vi "SetOpenedChannels.vi"(7 "Slot":T1, 8 "Error In":errorcluster, 9 "All?":bool, 10 "Channels":bool[](array[boolean]), 11 "Keithley 7001 In":refnum<visa-resource-name>) -> (0 "Error Out":errorcluster, 3 "Keithley 7001 Out":refnum<visa-resource-name>)   [LabVIEW 2012, in "Keithley-7001.lvlib"]
uses:
  Keithley-7001.lvlib
  Controls/Slot.ctl
panel:
  # "33"
  # "34"
  # "35"
  # "1"
  # "2"
  # "3"
  # "4"
  # "5"
  # "6"
  # "7"
  # "8"
  # "9"
  # "10"
  # "11"
  # "12"
  # "13"
  # "14"
  # "15"
  # "16"
  # "17"
  # "18"
  # "19"
  # "20"
  # "21"
  # "22"
  # "23"
  # "24"
  # "25"
  # "26"
  # "27"
  # "28"
  # "29"
  # "30"
  # "31"
  # "32"
  # "36"
  # "37"
  # "38"
  # "39"
  # "40"
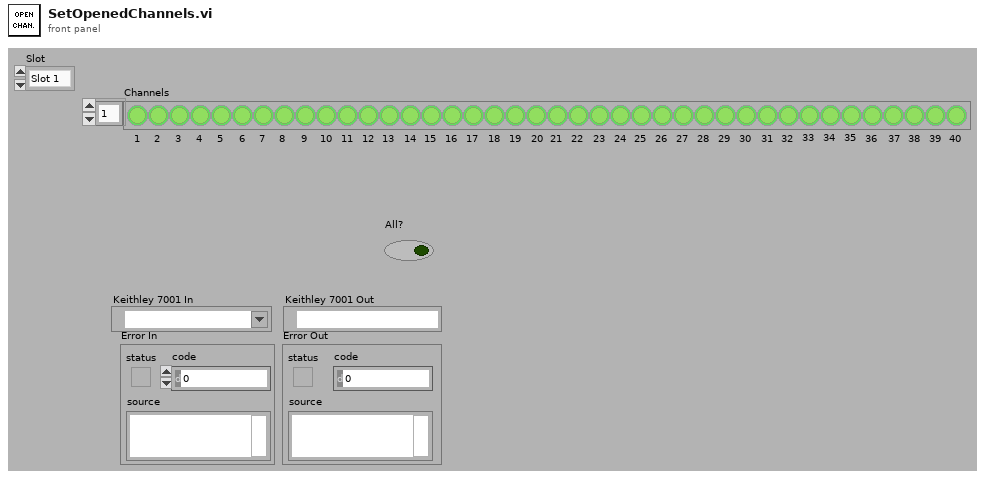
[diagram p1: front panel]
types:
  T1 = typedef "Keithley-7001.lvlib/Slot.ctl" = enum16{"Slot 1", "Slot 2"}
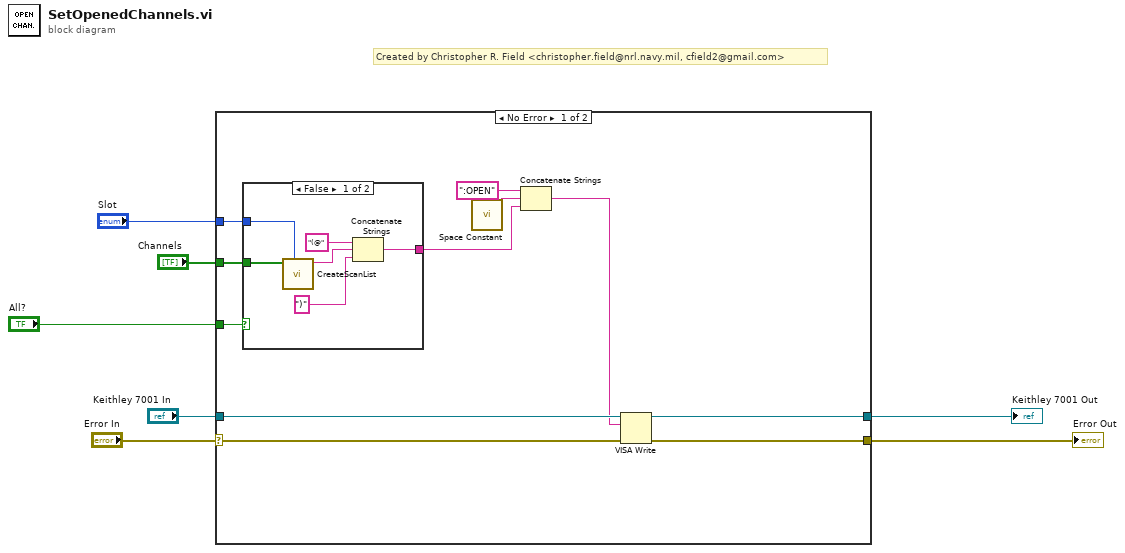
[diagram p0: block diagram]
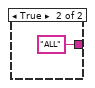
[diagram p2: hidden frame]
diagram:
  # "Created by Christopher R. Field <christopher.field@nrl.navy.mil, cfield2@gmail.com>"
  n1 = case shown="No Error" "Error In" {
    selector: "Error In" -> [w11 w26]
    tunnel: "Keithley 7001 In" -> [w18 w27]
    tunnel: [w17 w27] -> w6
    tunnel: [w16 w26] -> w5
    tunnel: "Channels" -> [w14 _]
    tunnel: "All?" -> [w9 _]
    tunnel: "Slot" -> [w8 _]
    frame No Error {
      n2 = case shown="False" w9 {
        tunnel: w14 -> [w24 _]
        tunnel: [w20 "ALL"] -> w10
        tunnel: w8 -> [w19 _]
        frame False {
          n3 = call "CreateScanList.vi"("Slot"=w19, "Channels"=w24) -> ("Channel List"=w22:string)  [unwired: 9 in]
          n4 = Concatenate Strings("(@", w22, ")" ("string")) -> (w20:string)
        }
        frame True {
        }
      }
      n5 = call <vilib>:"Space Constant.vi"() -> ("String"=w12:string)
      n6 = Concatenate Strings(":OPEN", w12, w10) -> (w13:string)
      n7 = VISA Write(VISA resource name=w18, write buffer=w13, error in (no error)=w11) -> (VISA resource name out=w17:refnum<visa-resource-name>, error out=w16:errorcluster)  [unwired: 1 out]
    }
    frame Error {
    }
  }
  "Keithley 7001 Out" <- w6
  "Error Out" <- w5
